vi "16_DC Motor_PID_test.vi"() -> ()   [LabVIEW 2018]
uses:
  <userlib>/KNR OS 4.0 LabVIEW Toolkit/Type Definition/Resource.ctl
  <userlib>/KNR OS 4.0 LabVIEW Toolkit/Type Definition/DC Motor Port.ctl
panel:
  in  "Port":T1=4 items=["DS1"=4, "DS2"=5, "DS3"=6, "DS4"=7]
  out "Velocity (cm/sec) Chart":dbl(graph)
  out "Speed (+-100%)":dbl
  in  "Desire Velosity (cm/sec)":dbl(slide) scale=0.0..200.0
  in  "Kd":dbl(slide) scale=0.0..0.02
  in  "Ki":dbl(slide) scale=0.0..0.2
  in  "Kp":dbl(slide) scale=0.0..1.0
  in  "IP":string(combo)="172.22.11.2"
  in  "Resource":T2=enum."KNRm_DDDD"
  in  "stop":bool
  in  "Enable Motor":bool
  out "Position cm":dbl
  out "Velocity (cm/sec)":dbl
  in  "Reverse?":bool
  in  "Reset":bool
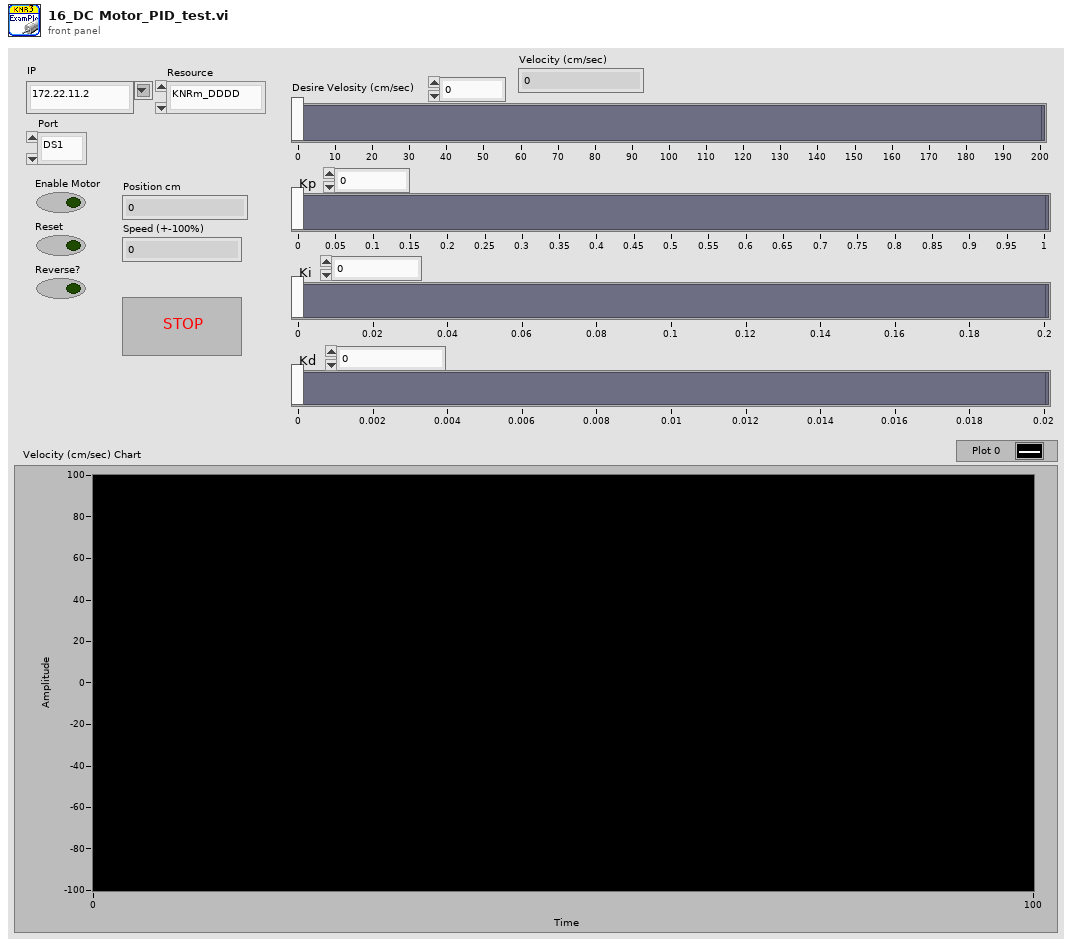
[diagram p1: front panel]
types:
  T1 = typedef "DC Motor Port.ctl" = u16
  T2 = typedef "Resource.ctl" = enum16{"KNRm_DDRC", "KNRm_DDDD", "KNRm_DDDR", "KNRm_DDDC", "KNR", "KNRm_neww"}
  T3 = typedef "KNR3 Reference.ctl" = cluster{"FPGA Session":refnum<class "FPGA Interface Base.lvclass">, "Resource":T2}
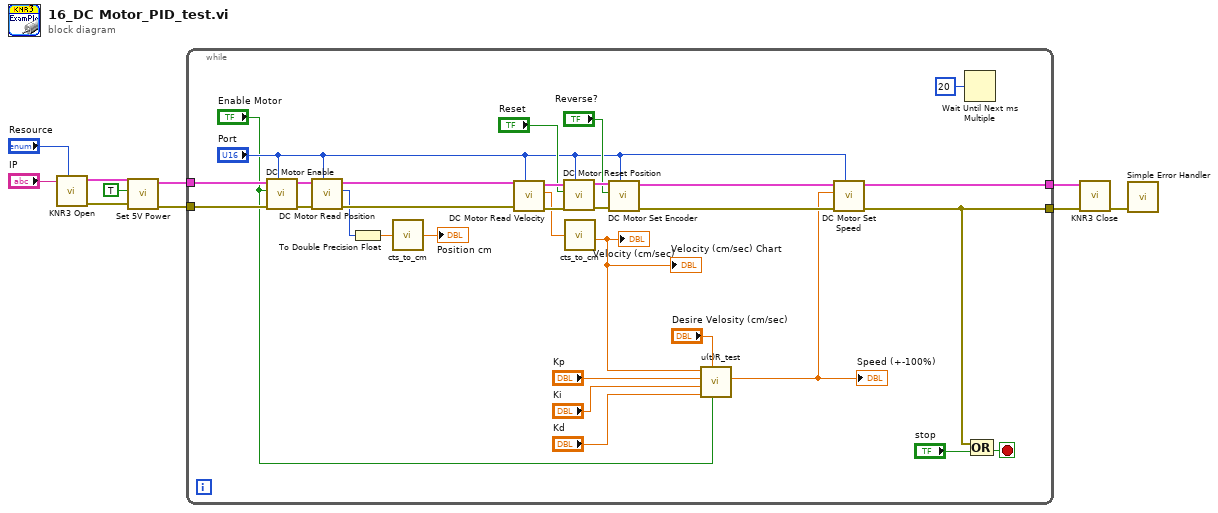
[diagram p0: block diagram]
diagram:
  n1 = call <userlib>:"KNR3 Open.vi"("Resource"="Resource", "IP"="IP") -> ("error out"=w4:errorcluster, "KNR out"=w6:T3)  [unwired: 8 in]
  n2 = call <userlib>:"Set 5V Power.vi"("error in (no error)"=w4, "5V Power(T)"=TRUE ("5V Power"), "KNR in"=w6) -> ("error out"=w8:errorcluster, "KNR out"=w9:T3)  [unwired: 7 in]
  n3 = while {
    tunnel: w9 -> [w41]
    tunnel: w8 -> [w40]
    tunnel: [w19] -> w2
    tunnel: [w18] -> w1
    stop <- w38 stop-if-true
    n4 = call <userlib>:"DC Motor Enable.vi"("Port (DS1)"="Port", "error in (no error)"=w40, "Enable Motor(F)"="Enable Motor", "KNR in"=w41) -> ("error out"=w23:errorcluster, "KNR out"=w24:T3)  [unwired: 6 in]
    n5 = call <userlib>:"DC Motor Read Position.vi"("Port (DS1)"="Port", "error in (no error)"=w23, "KNR in"=w24) -> ("error out"=w35:errorcluster, "Position"=w26:i32, "KNR out"=w36:T3)  [unwired: 6 in]
    n6 = To Double Precision Float(number=w26) -> (double precision float=w25:dbl)
    n7 = call "cts_to_cm.vi"("cts"=w25) -> ("cm"=→"Position cm":dbl)
    n8 = call <userlib>:"DC Motor Read Velocity.vi"("Port (DS1)"="Port", "error in (no error)"=w35, "KNR in"=w36) -> ("error out"=w31:errorcluster, "Velocity (cts/sec)"=w30:dbl, "KNR out"=w34:T3)  [unwired: 6 in]
    n9 = call <userlib>:"DC Motor Reset Position.vi"("Port (DS1)"="Port", "error in (no error)"=w31, "Reset(F)"="Reset", "KNR in"=w34) -> ("error out"=w32:errorcluster, "KNR out"=w33:T3)  [unwired: 6 in]
    n10 = call "cts_to_cm.vi"("cts"=w30) -> ("cm"=w12:dbl)
    "Velocity (cm/sec)" <- w12
    "Velocity (cm/sec) Chart" <- w12
    n11 = call <userlib>:"DC Motor Set Encoder.vi"("Port (DS1)"="Port", "error in (no error)"=w32, "Reverse?(F)"="Reverse?", "KNR in"=w33) -> ("error out"=w21:errorcluster, "KNR out"=w22:T3)  [unwired: 6 in]
    n12 = call "u(t)R_test.vi"("enable"="Enable Motor", "Desire Velosity"="Desire Velosity (cm/sec)", "Kd"="Kd", "Ki"="Ki", "Kp"="Kp", "Velocity"=w12) -> ("u(t)"=w13:dbl)  [unwired: 5 in]
    "Speed (+-100%)" <- w13
    n13 = call <userlib>:"DC Motor Set Speed.vi"("Port (DS1)"="Port", "error in (no error)"=w21, "Speed (+-100%)"=w13, "KNR in"=w22) -> ("error out"=w18:errorcluster, "KNR out"=w19:T3)  [unwired: 6 in]
    n14 = Wait Until Next ms Multiple(millisecond multiple=u32 20) -> ()  [unwired: 1 out]
    n15 = Compound Arithmetic op=OR(w18, "stop") -> (w38:bool)
  }
  n16 = call <userlib>:"KNR3 Close.vi"("error in (no error)"=w1, "KNR in"=w2) -> ("error out"=w7:errorcluster)  [unwired: 9 in]
  n17 = call <vilib>:"Simple Error Handler.vi"("error in (no error)"=w7) -> ()  [unwired: 4 in, 5 out]
